vi "Graphics-LTRB to WHCM (DBL).vi"(7 "LTRB":T1) -> (0 "Middle":dbl, 2 "Center":dbl, 3 "Height":dbl, 5 "Width":dbl)   [LabVIEW 2015]
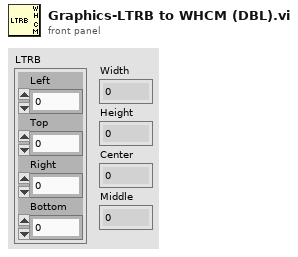
[diagram p1: front panel]
types:
  T1 = cluster{"Left":dbl, "Top":dbl, "Right":dbl, "Bottom":dbl}
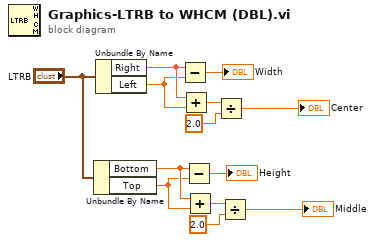
[diagram p0: block diagram]
diagram:
  n1 = Unbundle By Name("LTRB") -> ("Bottom"=w7:dbl, "Top"=w6:dbl)
  n2 = Unbundle By Name("LTRB") -> ("Right"=w13:dbl, "Left"=w12:dbl)
  n3 = Subtract(x=w13, y=w12) -> (x-y=→"Width":dbl)
  n4 = Add(x=w13, y=w12) -> (x+y=w11:dbl)
  n5 = Subtract(x=w7, y=w6) -> (x-y=→"Height":dbl)
  n6 = Add(x=w7, y=w6) -> (x+y=w5:dbl)
  n7 = Divide(x=w11, y=2.0) -> (x/y=→"Center":dbl)
  n8 = Divide(x=w5, y=2.0) -> (x/y=→"Middle":dbl)
